vi "getDAQmxTaskRef.vi"(8 "error in (no error)":errorcluster, 11 "niDAQmxDO.lvclass in":refnum<class "niDAQmxDO.lvclass">) -> (0 "error out":errorcluster, 2 "DAQmx Task Ref":refnum<k21>, 3 "niDAQmxDO.lvclass out":refnum<class "niDAQmxDO.lvclass">)   [LabVIEW 2009, in "Hardware.lvlib" / "Channels.lvlib" / "niDAQmxDO.lvclass"]
uses:
  niDAQmxDO.lvclass
  niDAQmxDO.lvclass/niDAQmxDO.ctl
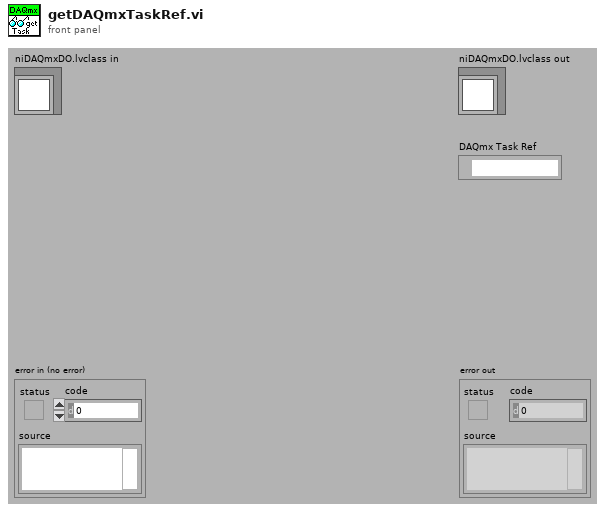
[diagram p1: front panel]
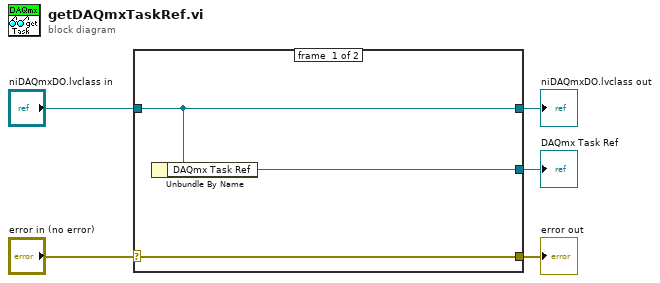
[diagram p0: block diagram]
diagram:
  n1 = case shown="No Error" "error in (no error)" {
    selector: "error in (no error)" -> [w8 w9]
    tunnel: [w8 w9] -> w4
    tunnel: [w7 w10] -> w2
    tunnel: "niDAQmxDO.lvclass in" -> [w7 w10]
    tunnel: [w6 _] -> w1
    frame #0 {
      n2 = Unbundle By Name(w7) -> ("DAQmx Task Ref"=w6:refnum<k21>)
    }
    frame #1 {
    }
  }
  "error out" <- w4
  "niDAQmxDO.lvclass out" <- w2
  "DAQmx Task Ref" <- w1
